vi "Cx Gamma.vi"(11 "z":cdb) -> (3 "g(z)":cdb format="%#_15g")   [LabVIEW 2010, in "NI_Gmath.lvlib"]
uses:
  NI_Gmath.lvlib
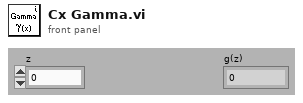
[diagram p1: front panel]
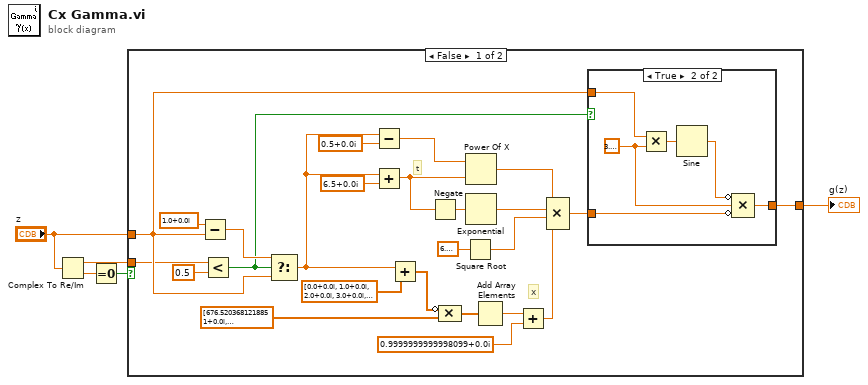
[diagram p0: block diagram]
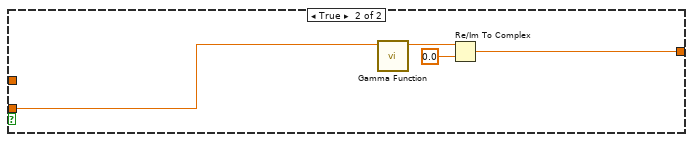
[diagram p3: hidden frame]
diagram:
  n1 = Complex To Re/Im(x + iy="z") -> (x=w1:dbl, y=w3:dbl)
  n2 = Equal To 0?(x=w3) -> (x = 0?=w2:bool)
  n3 = case shown="False" w2 {
    tunnel: "z" -> [w16 _]
    tunnel: [w15 w38] -> w5
    tunnel: w1 -> [w14 w41]
    frame False {
      # "x"
      # "t"
      n4 = Subtract(x=cdb 1.0+0.0i ("y"), y=w16) -> (x-y=w28:cdb)
      n5 = Less?(x=w14, y=0.5) -> (x < y?=w18:bool)
      n6 = Select(t=w28, s=w18, f=w16) -> (s? t:f=w13:cdb)
      n7 = Subtract(x=w13, y=cdb 0.5+0.0i) -> (x-y=w24:cdb)
      n8 = Add(x=w13, y=cdb 6.5+0.0i) -> (x+y=w22:cdb)
      n9 = Add(x=w13, y=cdb[] [0.0+0.0i, 1.0+0.0i, 2.0+0.0i, 3.0+0.0i, 4.0+0.0i, 5.0+0.0i, 6.0+0.0i, 7.0+0.0i] ("Ramp Pattern")) -> (x+y=w9:cdb[])
      n10 = Negate(x=w22) -> (-x=w23:cdb)
      n11 = Compound Arithmetic op=MULTIPLY(invert w9, cdb[] [676.5203681218851+0.0i, -1259.1392167224028+0.0i, 771.3234287776531+0.0i, -176.6150291621406+0.0i, 12.507343278686905+0.0i, -0.13857109526572012+0.0i, 9.984369578019572e-06+0.0i, 1.5056327351493116e-07+0.0i] ("array w/ subset deleted")) -> (w12:cdb[])
      n12 = Square Root(x=6.283185307179586) -> (sqrt(x)=w21:dbl)
      n13 = Power Of X(1:w22, 2:w24) -> (0:w20:cdb)
      n14 = Exponential(1:w23) -> (0:w19:cdb)
      n15 = Add Array Elements(numeric array=w12) -> (sum=w11:cdb)
      n16 = Add(x=w11, y=cdb 0.9999999999998099+0.0i ("deleted portion")) -> (x+y=w10:cdb)
      n17 = Compound Arithmetic op=MULTIPLY(w20, w19, w21, w10) -> (w17:cdb)
      n18 = case shown="True" w18 {
        tunnel: w17 -> [w31 w33]
        tunnel: [w31 w32] -> w15
        tunnel: w16 -> [_ w37]
        frame False {
        }
        frame True {
          w34 = 3.141592653589793
          n19 = Multiply(x=w37, y=w34) -> (x*y=w36:cdb)
          n20 = Sine(x=w36) -> (sin(x)=w35:cdb)
          n21 = Compound Arithmetic op=MULTIPLY(invert w35, w34, invert w33) -> (w32:cdb)
        }
      }
    }
    frame True {
      n22 = call "Gamma Function.vi"("x"=w41) -> ("g(x)"=w40:dbl)  [unwired: 10 out]
      n23 = Re/Im To Complex(1:0.0 ("y"), 2:w40) -> (0:w38:cdb)
    }
  }
  "g(z)" <- w5
